vi "Acq-module-5781.vi"(5 "IntermediateFIFO":refnum<k21>="FIFO0", 7 "AI Cluster":T2={"FPGA AI1"="IO Module\\AI 1 Data N", "FPGA AI1 2"="IO Module\\AI 1 Data N"}, 8 "NumChannels":T1, 9 "SamplingRate0":u16, 11 "Cluster in":T4={0, 0, 0, 0, 0, 0, 0, TRUE, TRUE, 0, 0, 0}) -> (1 "Analog Out Cluster":T3, 3 "cluster out":T4)   [LabVIEW 2013]
uses:
  N Channels 5781.ctl
  <vilib>/rvi/DataTransferAndStorage/Container/Common/niFpgaContainerExecOnDevCompGetState.vi
  <vilib>/rvi/FIFO/Fifo_Resource/nirvififoEmulationWriteFpgaImpl.vi
  <vilib>/rvi/DataTransferAndStorage/Container/Common/niFpgaContainerGetUniqueNameForEmu.vi
  <vilib>/rvi/interface/RandomDataEmulation/nirviRandomDataFPGAFIFO.vi
  <vilib>/rvi/interface/RandomDataEmulation/niFpgaRandomDataHandleErrors.vi
  <vilib>/rvi/eio/common/nirviEmuReportErrorAndStop.vi
  <vilib>/rvi/eio/common/nirviEmuTemplateMethod_errors.vi
  <vilib>/rvi/DataTransferAndStorage/Container/XNode/niFpgaContainer.xnode
  <vilib>/rvi/FIFO/Fifo_Resource/niFpgaFifoEmulationRefIn.vi
  <vilib>/eio/EIONode/EIONode.xnode
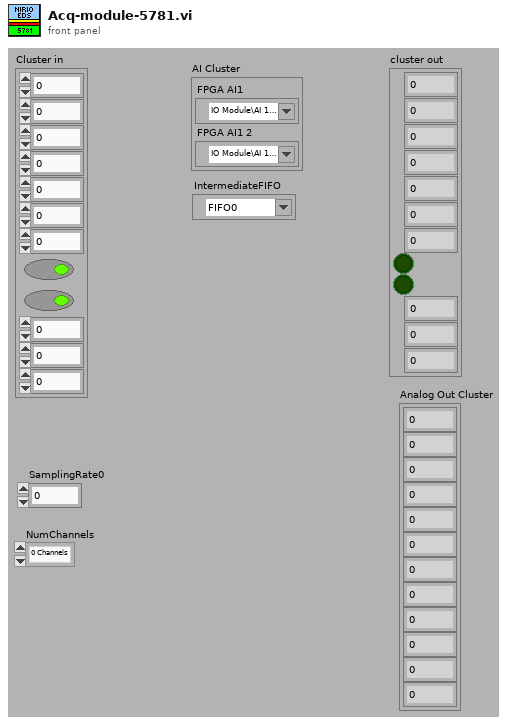
[diagram p1: front panel]
types:
  T1 = typedef "N Channels 5781.ctl" = enum16{"0 Channels", "1 Channels", "2 Channels"}
  T2 = cluster{"FPGA AI1":refnum<k21>, "FPGA AI1 2":refnum<k21>}
  T3 = cluster{i16, i16, i16, i16, i16, i16, i16, i16, i16, i16, i16, i16}
  T4 = cluster{u16, u16, u64, u64, u64, u64, i16, bool, bool, u64, u16, u16}
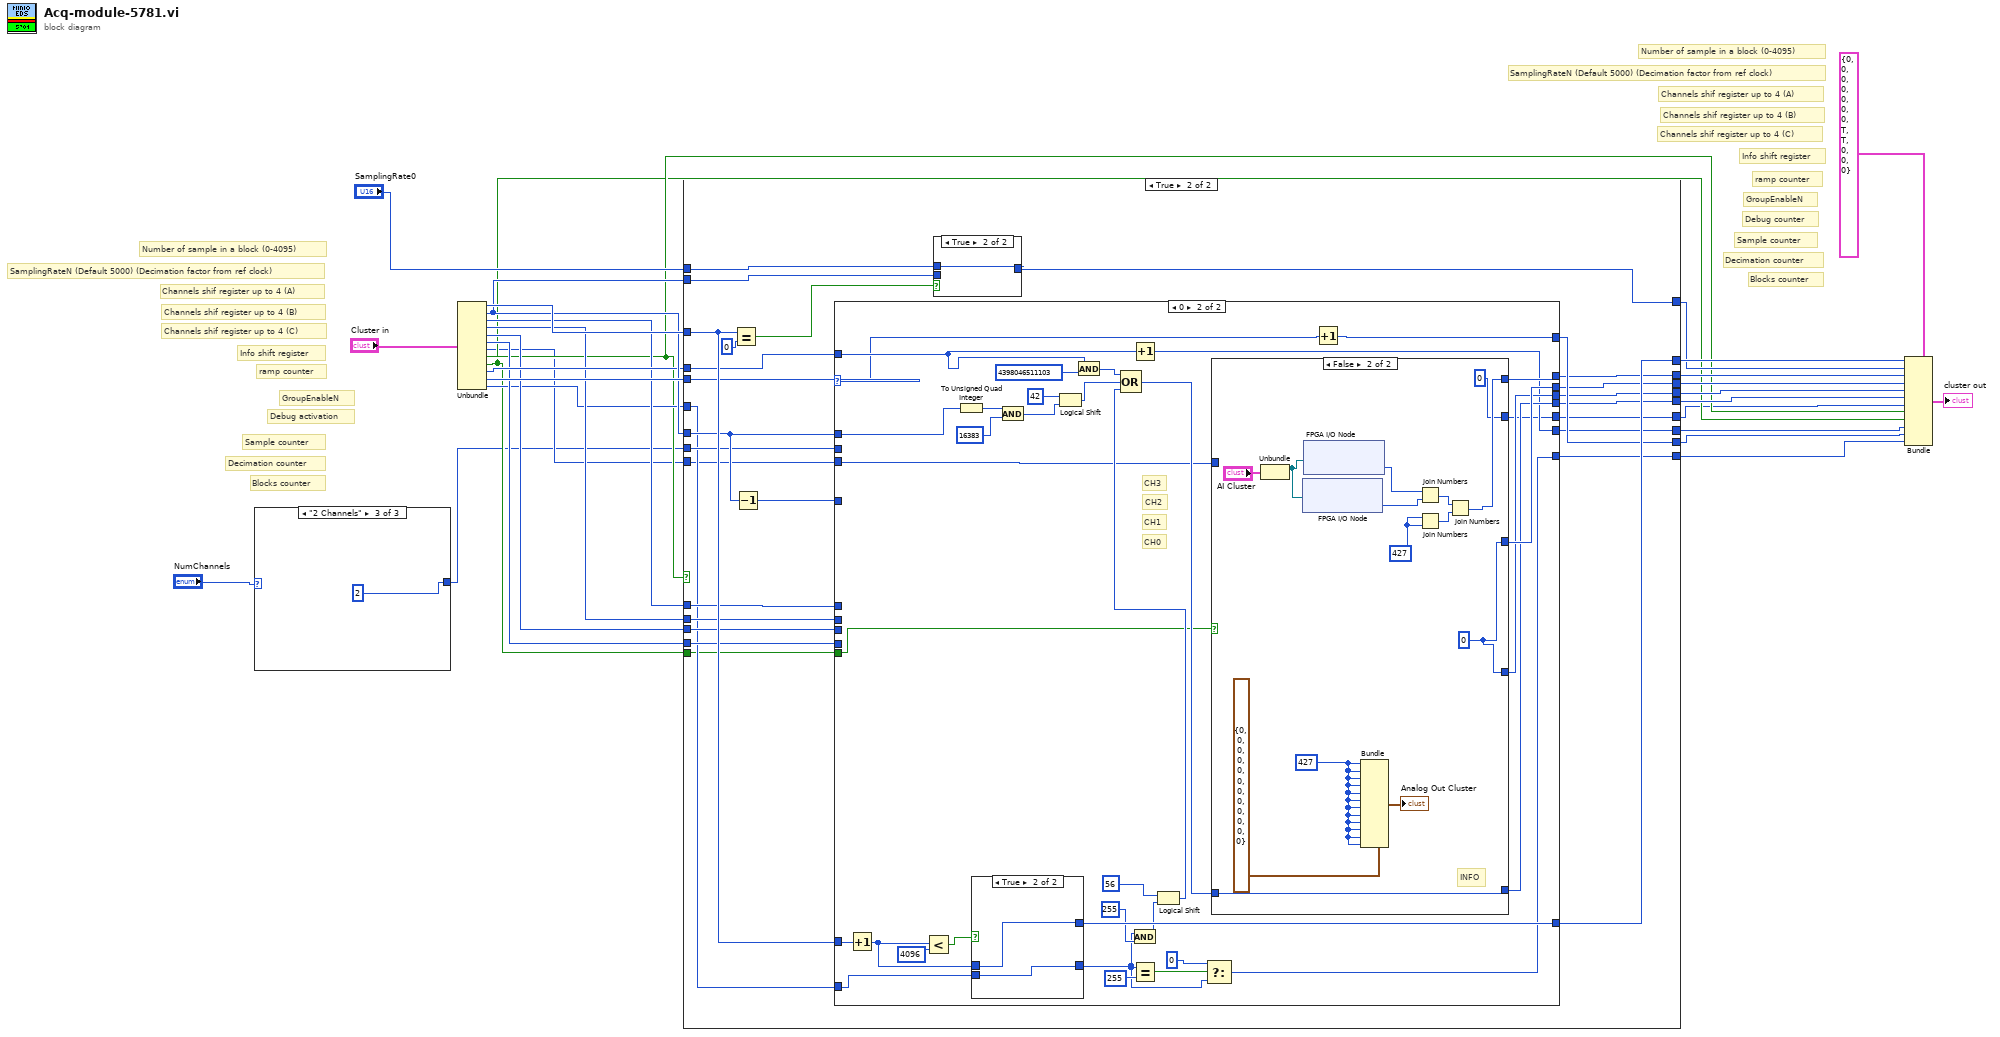
[diagram p0: block diagram]
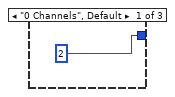
[diagram p2: hidden frame]
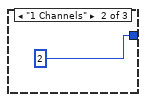
[diagram p3: hidden frame]
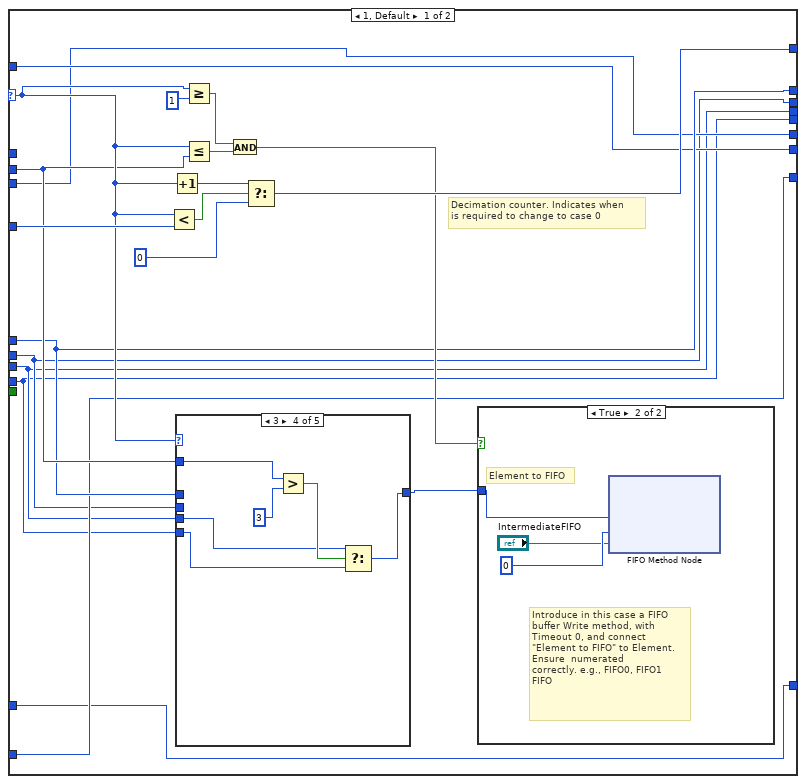
[diagram p5: hidden frame]
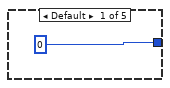
[diagram p7: hidden frame]
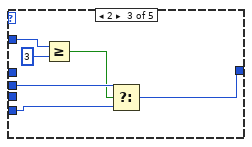
[diagram p9: hidden frame]
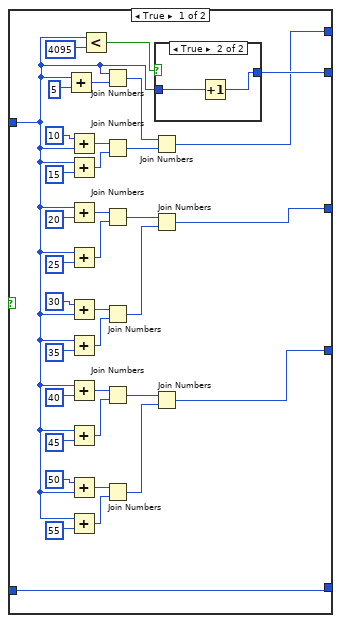
[diagram p11: hidden frame]
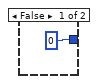
[diagram p12: hidden frame]
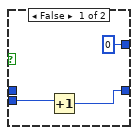
[diagram p13: hidden frame]
diagram:
  # "Blocks counter"
  # "Decimation counter"
  # "Blocks counter"
  # "Sample counter"
  # "Debug counter"
  # "ramp counter"
  # "Info shift register"
  # "Channels shif register up to 4 (C)"
  # "Channels shif register up to 4 (B)"
  # "Channels shif register up to 4 (A)"
  # "SamplingRateN (Default 5000) (Decimation factor from ref clock)"
  # "Number of sample in a block (0-4095)"
  # "GroupEnableN"
  # "Decimation counter"
  # "Sample counter"
  # "Debug activation"
  # "ramp counter"
  # "Info shift register"
  # "Channels shif register up to 4 (C)"
  # "Channels shif register up to 4 (B)"
  # "Channels shif register up to 4 (A)"
  # "SamplingRateN (Default 5000) (Decimation factor from ref clock)"
  # "Number of sample in a block (0-4095)"
  # "GroupEnableN"
  n1 = case shown="\"2 Channels\"" "NumChannels" {
    tunnel: [u8 2 ("Number of words") u8 2 ("Number of words") u8 2 ("Number of words")] -> w2
    frame "0 Channels", Default {
    }
    frame "1 Channels" {
    }
    frame "2 Channels" {
    }
  }
  n2 = Unbundle("Cluster in") -> (w28:u16, w15:u16, w12:u64, w11:u64, w10:u64, w9:u64, w4:i16, w6:bool, w5:bool, w14:u64, w21:u16, w8:u16)
  n3 = case shown="True" w6 {
    tunnel: w28 -> [w39 w64]
    tunnel: "SamplingRate0" -> [_ w67]
    tunnel: w15 -> [w40 w65]
    tunnel: [w39 w63] -> w25
    tunnel: [w40 w62] -> w24
    tunnel: w15 -> [_ w61]
    tunnel: w2 -> [_ w59]
    tunnel: w21 -> [w41 w58]
    tunnel: [w41 w57] -> w20
    tunnel: [w38 w56] -> w19
    tunnel: [w37 w55] -> w18
    tunnel: [w36 w54] -> w17
    tunnel: [w35 w53] -> w16
    tunnel: w14 -> [w34 w52]
    tunnel: [w34 w51] -> w13
    tunnel: w12 -> [w38 w50]
    tunnel: w11 -> [w37 w49]
    tunnel: w10 -> [w36 w48]
    tunnel: w9 -> [w35 w47]
    tunnel: w8 -> [w33 w46]
    tunnel: [w33 w45] -> w7
    tunnel: w5 -> [_ w44]
    tunnel: w4 -> [w32 w43]
    tunnel: [w32 w42] -> w3
    frame False {
    }
    frame True {
      n4 = Equal?(x=w64, y=u16 0) -> (x = y?=w66:bool)
      n5 = Decrement(x=w61) -> (x-1=w60:u16)
      n6 = case shown="0" w58 {
        selector: w58 -> [w80 w108]
        tunnel: w64 -> [w73 w141]
        tunnel: [w73 w137] -> w63
        tunnel: w61 -> [_ w134]
        tunnel: w60 -> [w83 _]
        tunnel: w59 -> [w79 _]
        tunnel: [w82 w107] -> w57
        tunnel: [w77 w121] -> w56
        tunnel: [w71 w120] -> w55
        tunnel: [w70 w119] -> w54
        tunnel: [w69 w118] -> w53
        tunnel: w52 -> [w75 w116]
        tunnel: [w75 w115] -> w51
        tunnel: w50 -> [w77 _]
        tunnel: w49 -> [w71 _]
        tunnel: w48 -> [w70 _]
        tunnel: w47 -> [w69 _]
        tunnel: w46 -> [w74 w114]
        tunnel: [w74 w113] -> w45
        tunnel: w44 -> [_ w112]
        tunnel: w43 -> [w72 w111]
        tunnel: [w72 w110] -> w42
        frame 1, Default {
          # "Decimation counter. Indicates when \nis required to change to case 0"
          n7 = Less?(x=w80, y=w83) -> (x < y?=w76:bool)
          n8 = Increment(x=w80) -> (x+1=w88:u16)
          n9 = case shown="3" w80 {
            tunnel: [u64 0 ("Element") w93 w96 w100 w106] -> w81
            tunnel: w77 -> [_ w93 _ _ _]
            tunnel: w71 -> [_ _ w99 _ _]
            tunnel: w70 -> [_ _ _ w102 _]
            tunnel: w69 -> [_ _ w95 w101 w106]
            tunnel: w79 -> [_ _ w98 w105 _]
            frame Default {
            }
            frame 1 {
            }
            frame 2 {
              n10 = Greater Or Equal?(x=w98, y=u8 3) -> (x >= y?=w94:bool)
              n11 = Select(t=w99, s=w94, f=w95) -> (s? t:f=w96:u64)
            }
            frame 3 {
              n12 = Greater?(x=w105, y=u8 3) -> (0:w103:bool)
              n13 = Select(t=w102, s=w103, f=w101) -> (s? t:f=w100:u64)
            }
            frame 4 {
            }
          }
          n14 = Greater Or Equal?(x=w80, y=u16 1) -> (x >= y?=w85:bool)
          n15 = Less Or Equal?(x=w80, y=w79) -> (x <= y?=w84:bool)
          n16 = And(x=w85, y=w84) -> (x .and. y?=w78:bool)
          n17 = Select(t=w88, s=w76, f=u16 0) -> (s? t:f=w82:u16)
          n18 = case shown="True" w78 {
            tunnel: w81 -> [_ w91]
            frame False {
            }
            frame True {
              # "Element to FIFO"
              # "Introduce in this case a FIFO buffer Write method, with Timeout 0, and connect \"Element to FIFO\" to Element. Ensure  numerated\ncorrectly. e.g., FIFO0, FIFO1 \nFIFO"
              n19 = xnode ("FIFO Method Node")("Element"=w91, "Timeout"=0, "FIFO In"="IntermediateFIFO") -> ()  [unwired: 2 out]
            }
          }
        }
        frame 0 {
          # "CH0"
          # "CH1"
          # "CH2"
          # "CH3"
          n20 = Increment(x=w141) -> (x+1=w138:u16)
          n21 = Less?(x=w138, y=u16 4096) -> (x < y?=w139:bool)
          n22 = To Unsigned Quad Integer(1:w134) -> (0:w136:u64)
          n23 = case shown="True" w139 {
            tunnel: w138 -> [_ w199]
            tunnel: [u16 0 w199] -> w137
            tunnel: w114 -> [w196 w198]
            tunnel: [w195 w198] -> w109
            frame False {
              n24 = Increment(x=w196) -> (x+1=w195:u16)
            }
            frame True {
            }
          }
          n25 = And(x=w136, y=i16 16383) -> (x .and. y?=w133:u64)
          n26 = Logical Shift(y=i8 42, x=w133) -> (x << y=w129:u64)
          n27 = And(x=w116, y=u64 4398046511103) -> (x .and. y?=w130:u64)
          n28 = Increment(x=w116) -> (x+1=w115:u64)
          n29 = And(x=w109, y=u64 255) -> (x .and. y?=w127:u64)
          n30 = Equal?(x=w109, y=u16 255) -> (x = y?=w124:bool)
          n31 = Logical Shift(y=i8 56, x=w127) -> (x << y=w122:u64)
          n32 = Compound Arithmetic op=OR(w130, w129, w122) -> (w117:u64)
          n33 = Select(t=u16 0, s=w124, f=w109) -> (s? t:f=w113:u16)
          n34 = case shown="False" w112 {
            tunnel: [w145 w194] -> w121
            tunnel: [w144 w188] -> w120
            tunnel: [w143 w188] -> w119
            tunnel: [w142 w193] -> w118
            tunnel: w117 -> [w142 w193]
            tunnel: w111 -> [w147 _]
            tunnel: [w146 i16 0] -> w110
            frame True {
              n35 = Add(x=w147, y=i16 5) -> (x+y=w174:i16)
              n36 = Add(x=i16 10, y=w147) -> (x+y=w172:i16)
              n37 = Add(x=w147, y=i16 15) -> (x+y=w170:i16)
              n38 = Add(x=w147, y=i16 20) -> (x+y=w159:i16)
              n39 = Add(x=w147, y=i16 25) -> (x+y=w164:i16)
              n40 = Add(x=i16 30, y=w147) -> (x+y=w162:i16)
              n41 = Add(x=w147, y=i16 35) -> (x+y=w160:i16)
              n42 = Add(x=w147, y=i16 40) -> (x+y=w149:i16)
              n43 = Add(x=w147, y=i16 45) -> (x+y=w154:i16)
              n44 = Add(x=i16 50, y=w147) -> (x+y=w152:i16)
              n45 = Add(x=w147, y=i16 55) -> (x+y=w150:i16)
              n46 = Less?(x=w147, y=i16 4095) -> (x < y?=w168:bool)
              n47 = Join Numbers(hi=w147, lo=w174) -> ((hi.lo)=w177:u32)
              n48 = Join Numbers(hi=w172, lo=w170) -> ((hi.lo)=w176:u32)
              n49 = Join Numbers(hi=w159, lo=w164) -> ((hi.lo)=w167:u32)
              n50 = Join Numbers(hi=w162, lo=w160) -> ((hi.lo)=w166:u32)
              n51 = Join Numbers(hi=w149, lo=w154) -> ((hi.lo)=w157:u32)
              n52 = Join Numbers(hi=w152, lo=w150) -> ((hi.lo)=w156:u32)
              n53 = Join Numbers(hi=w177, lo=w176) -> ((hi.lo)=w145:u64)
              n54 = Join Numbers(hi=w167, lo=w166) -> ((hi.lo)=w144:u64)
              n55 = Join Numbers(hi=w157, lo=w156) -> ((hi.lo)=w143:u64)
              n56 = case shown="True" w168 {
                tunnel: w147 -> [_ w180]
                tunnel: [i16 0 w179] -> w146
                frame False {
                }
                frame True {
                  n57 = Increment(x=w180) -> (x+1=w179:i16)
                }
              }
            }
            frame False {
              w183 = u16 427 ("hi")
              w188 = 0 ("Timeout")
              w190 = i16 427
              # "INFO"
              n58 = Unbundle("AI Cluster") -> ("FPGA AI1"=w181:refnum<k21>)  [unwired: 1 out]
              n59 = xnode "FPGA I/O Node"("FPGA I/O In"=w181) -> ("I/O Item"=w184:i16)  [unwired: 1 out]
              n60 = xnode "FPGA I/O Node"("FPGA I/O In"=w181) -> ("I/O Item"=w185:i16)  [unwired: 1 out]
              n61 = Bundle(cluster=T3 {0, 0, 0, 0, 0, 0, 0, 0, 0, 0, 0, 0} ("Cluster 2"), w190, w190, w190, w190, w190, w190, w190, w190, w190, w190, w190, w190) -> (→"Analog Out Cluster":T3)
              n62 = Join Numbers(hi=w185, lo=w184) -> ((hi.lo)=w186:u32)
              n63 = Join Numbers(hi=w183, lo=w183) -> ((hi.lo)=w187:u32)
              n64 = Join Numbers(hi=w186, lo=w187) -> ((hi.lo)=w194:u64)
            }
          }
          n65 = Increment(x=w108) -> (x+1=w107:u16)
        }
      }
      n66 = case shown="True" w66 {
        tunnel: w67 -> [_ w201]
        tunnel: [w200 w201] -> w62
        tunnel: w65 -> [w200 _]
        frame False {
        }
        frame True {
        }
      }
    }
  }
  n67 = Bundle(cluster=T4 {0, 0, 0, 0, 0, 0, 0, TRUE, TRUE, 0, 0, 0} ("Cluster in"), w25, w24, w19, w18, w17, w16, w3, w6, w5, w13, w20, w7) -> (→"cluster out":T4)
